vi "VisionTrackingLabVeiwCode.vi"(0 "Image In":T1, 7 "error in":errorcluster) -> (20 "Image Out":T1, 27 "error out":errorcluster)   [LabVIEW 2016]
uses:
  <vilib>/vision/Image Controls.llb/IMAQ Image.ctl
  <vilib>/vision/Tracking.llb/IMAQ Object Tracking SessionType.ctl
  <vilib>/vision/Vision Assistant Utils.llb/IVA Object Tracking - Init Function.ctl
  <vilib>/vision/NI_Vision_Development_Module.lvlib
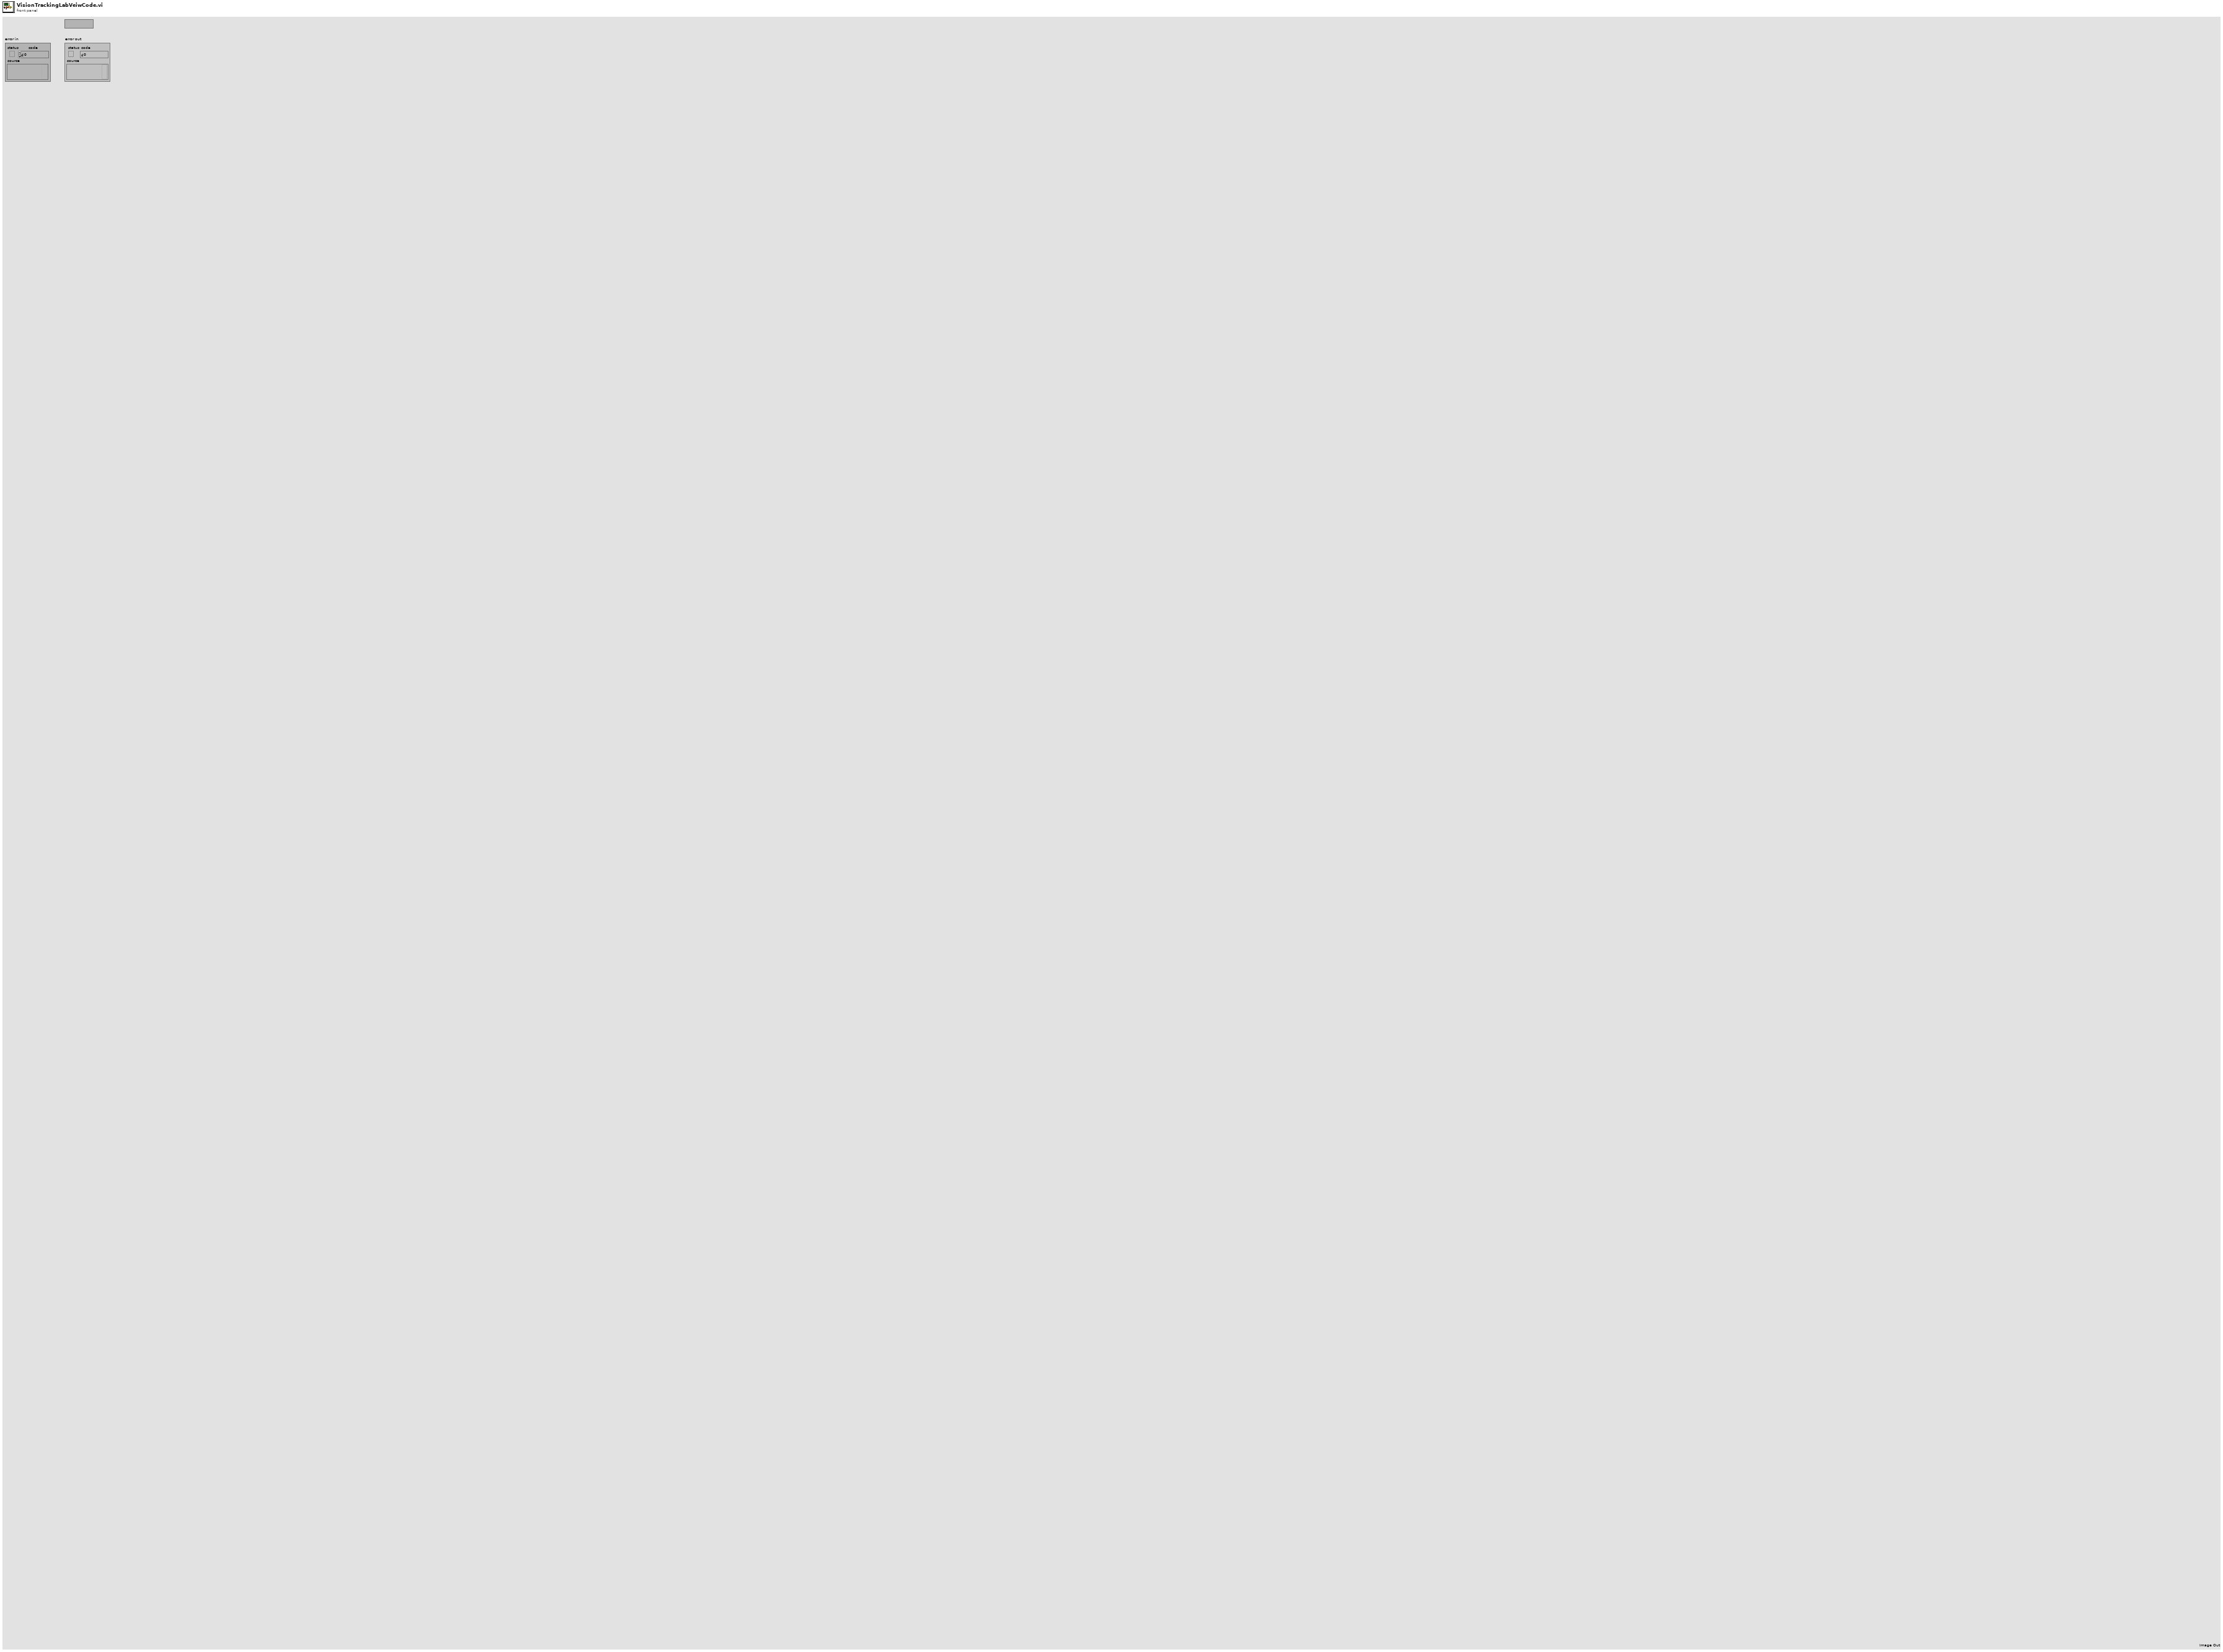
[diagram p1: front panel]
types:
  T1 = typedef "IMAQ Image.ctl" = refnum<image>
  T2 = cluster{"Number of Histogram Bins":i32, "Blending Parameter (%)":dbl, "Max Scale Change (%)":dbl, "Max Rotation Change":dbl, "Max Shape Change (%)":dbl, "Maximum Iterations":i32}
  T3 = typedef "IVA Object Tracking - Init Function.ctl" = enum16{"Init", "Get", "Set"}
  T4 = cluster{"Initial Position":cluster{"Source":enum16{"Constant", "Measure"}, "Point ID":cluster{"GUID":string, "Index":i32}, "Point":cluster{"x":sgl, "y":sgl}}, "Initial Angle":cluster{"Source":enum16{"Constant", "Measure"}, "Measure ID":cluster{"GUID":string, "Index":i32}, "Value":dbl}}[]
  T5 = typedef "IMAQ Object Tracking SessionType.ctl" = i32
  T6 = typedef "Image Type" = u32
  T7 = cluster{"Global Rectangle":i32[], "Contours":cluster{"ID":enum32{"External", "Internal"}, "Type":u32, "Coordinates":i32[]}[]}
  T8 = cluster{"Brightness":sgl, "Contrast":sgl, "Gamma":sgl}
  T9 = cluster{"Position":cluster{"x":sgl, "y":sgl}, "Angle":sgl, "Scale":sgl, "Score":sgl, "Bounding Box":cluster{"x":sgl, "y":sgl}[]}[]
  T10 = cluster{"Number of Histogram Bins":i32, "Blending Parameter (%)":dbl, "Maximum Iterations":i32}
  T11 = typedef "IMAQ Object Tracking Session.ctl" = refnum<k20>
  T12 = cluster{"Source":enum16{"Constant", "Measure"}, "Point ID":cluster{"GUID":string, "Index":i32}, "Point":cluster{"x":sgl, "y":sgl}}
  T13 = cluster{"Source":enum16{"Constant", "Measure"}, "Measure ID":cluster{"GUID":string, "Index":i32}, "Value":dbl}
  T14 = cluster{"Label":string, "Score":i32, "Angle":dbl, "Location":cluster{"X":dbl, "Y":dbl}, "Bounding Box":cluster{"X":dbl, "Y":dbl}[], "Object Found?":bool}[]
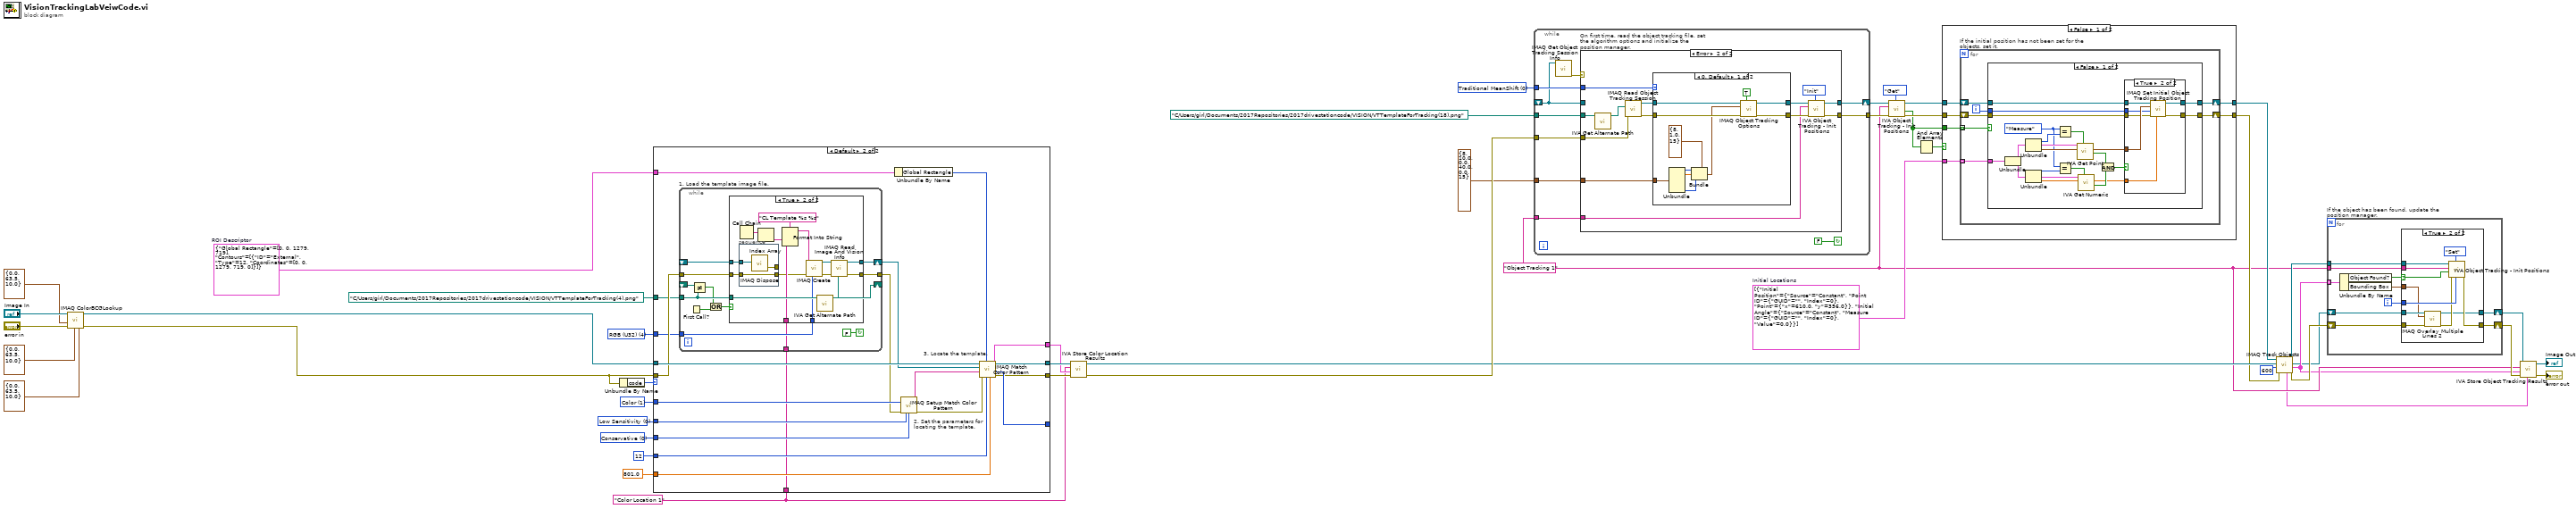
[diagram p0: block diagram]
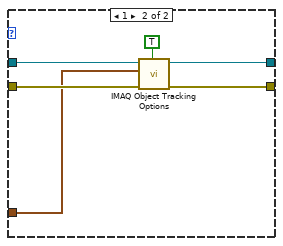
[diagram p7: hidden frame]
diagram:
  w6 = "Object Tracking 1" ("Step Name")
  w21 = T4 [{"Initial Position"={"Source"=enum."Constant", "Point ID"={"GUID"="", "Index"=0}, "Point"={"x"=610.0, "y"=356.0}}, "Initial Angle"={"Source"=enum."Constant", "Measure ID"={"GUID"="", "Index"=0}, "Value"=0.0}}]  # Initial Locations
  w23 = T5 0 items=["Traditional MeanShift", "Shape Adapted MeanShift"] ("Algorithm")
  w26 = "Color Location 1" ("Step Name")
  w34 = T6 4 items=["Grayscale (U8)", "Grayscale (I16)", "Grayscale (SGL)", "Complex (CSG)", "RGB (U32)", "HSL (U32)", "RGB (U64)"] ("Image Type")
  w36 = u32 0 items=["Conservative", "Balance", "Aggressive", "Very Aggressive"] ("Search Strategy")
  w37 = u32 0 items=["Low Sensitivity", "Medium Sensitivity", "High Sensitivity"] ("Color Sensitivity")
  w38 = u32 1 items=["Color and Shape", "Color", "Shape"] ("Match Feature Mode")
  w33 = T7 {"Global Rectangle"=[0, 0, 1279, 719], "Contours"=[{"ID"=enum."External", "Type"=12, "Coordinates"=[0, 0, 1279, 719, 0]}]}  # ROI Descriptor
  n1 = call "IMAQ ColorBCGLookup"("Blue BCG Values"=T8 {"Brightness"=0.0, "Contrast"=63.5, "Gamma"=10.0}, "Green BCG Values"=T8 {"Brightness"=0.0, "Contrast"=63.5, "Gamma"=10.0}, "error in (no error)"="error in", "Red BCG Values"=T8 {"Brightness"=0.0, "Contrast"=63.5, "Gamma"=10.0}, "Image Src"="Image In") -> ("error out"=w44:errorcluster, "Image Dst Out"=w32:T1)  [unwired: 2 in, 3 out]
  n2 = Unbundle By Name(w44) -> ("code"=w31:i32)
  n3 = case shown="Default" w31 {
    tunnel: sgl 801.0 ("Minimum Match Score") -> [_ w66]
    tunnel: 12 ("Number of Matches Requested") -> [_ w65]
    tunnel: [_ w64] -> _
    tunnel: w38 -> [_ w63]
    tunnel: w37 -> [_ w62]
    tunnel: w36 -> [_ w61]
    tunnel: path "C:/Users/girl/Documents/2017Repositories/2017drivestationcode/VISION/VTTemplateForTracking(4).png" ("File Path") -> [_ w53]
    tunnel: w34 -> [_ w52]
    tunnel: w44 -> [_ w54]
    tunnel: w33 -> [_ w58]
    tunnel: [_ w56] -> w27
    tunnel: w32 -> [w47 w55]
    tunnel: [w47 w55] -> w28
    tunnel: [_ w49] -> w29
    tunnel: w26 -> [_ w48]
    frame -1074396199, -1074396198 {
      # "Discard Coordinate System Error"
    }
    frame Default {
      # "3. Locate the template."
      # "2. Set the parameters for\nlocating the template."
      n4 = while "1. Load the template image file." {
        shift-right: [w78] -> w51
        shift-left: _ -> [w77]
        tunnel: [w75] -> w50
        tunnel: w54 -> [w74]
        tunnel: w53 -> [w70]
        tunnel: w52 -> [w73]
        tunnel: w48 -> [w72]
        shift-right: [w70] -> _
        shift-left: _ -> [w71]
        stop <- FALSE continue-if-true
        n5 = First Call?() -> (First Call?: T/F=w69:bool)
        n6 = Not Equal?(x=w71, y=w70) -> (x != y?=w68:bool)
        n7 = Or(x=w68, y=w69) -> (x .or. y?=w67:bool)
        n8 = case shown="True" w67 {
          tunnel: [w80 w93] -> w78
          tunnel: w77 -> [w80 w85]
          tunnel: [w79 w90] -> w75
          tunnel: w74 -> [w79 w84]
          tunnel: w73 -> [_ w89]
          tunnel: w72 -> [_ w86]
          tunnel: w70 -> [_ w82]
          frame False {
          }
          frame True {
            n9 = Call Chain() -> (call chain=w88:string[])
            n10 = stacked-sequence {
              tunnel: w85 -> [w98]
              tunnel: w84 -> [w97]
              tunnel: [w97] -> w83
              tunnel: [w96] -> _
              frame #0 {
                n11 = call "IMAQ Dispose"("Image"=w98) -> ("error out"=w96:errorcluster)  [unwired: 2 in, 3 out]
              }
            }
            n12 = Index Array(array=w88) -> (element=w87:string)  [unwired: 1 in]
            n13 = Format Into String(format string="CL Template %s %s" ("Image Name"), w87, w86) -> (resulting string=w95:string)  [unwired: 2 in, 1 out]
            n14 = call "IMAQ Create"("Image Name"=w95, "Image Type"=w89, "error in (no error)"=w83) -> ("New Image"=w92:T1, "error out"=w91:errorcluster)  [unwired: 1 in, 1 out]
            n15 = call <vilib>:"IVA Get Alternate Path.vi"("Path In"=w82) -> ("Path Out"=w81:path)  [unwired: 10 out]
            n16 = call "IMAQ Read Image And Vision Info"("File Path"=w81, "error in (no error)"=w91, "Image"=w92) -> ("error out"=w90:errorcluster, "Image Out"=w93:T1)  [unwired: 1 in, 6 out]
          }
        }
      }
      n17 = Unbundle By Name(w58) -> ("Global Rectangle"=w57:i32[])
      n18 = call "IMAQ Setup Match Color Pattern"("Match Feature Mode"=w63, "error in (no error)"=w50, "Color Sensitivity"=w62, "Search Strategy"=w61) -> ("Match Color Pattern Setup Data"=w60:string, "error out"=w59:errorcluster)  [unwired: 5 in, 5 out]
      n19 = call "IMAQ Match Color Pattern"("Minimum Match Score"=w66, "Number of Matches Requested"=w65, "Optional Rectangle"=w57, "error in (no error)"=w59, "Match Color Pattern Setup Data"=w60, "Template Image"=w51, "Image"=w55) -> ("error out"=w49:errorcluster, "Number of Matches"=w64:i32, "Matches"=w56:T9)  [unwired: 2 out]
    }
  }
  n20 = call <vilib>:"IVA Store Color Location Results.vi"("error in (no error)"=w29, "Matches"=w27, "Step Name"=w26, "Image in"=w28) -> ("error out"=w30:errorcluster, "Image dup"=w24:T1)  [unwired: 6 out]
  n21 = while {
    shift-right: [w108] -> w19
    shift-left: _ -> [w99]
    tunnel: path "C:/Users/girl/Documents/2017Repositories/2017drivestationcode/VISION/VTTemplateForTracking(18).png" ("Tracking Session File Path") -> [w106]
    tunnel: w30 -> [w105]
    tunnel: w23 -> [w104]
    tunnel: [w103] -> w16
    tunnel: T2 {"Number of Histogram Bins"=8, "Blending Parameter (%)"=10.0, "Max Scale Change (%)"=0.0, "Max Rotation Change"=40.0, "Max Shape Change (%)"=0.0, "Maximum Iterations"=15} ("Options") -> [w102]
    tunnel: w6 -> [w101]
    stop <- FALSE continue-if-true
    n22 = call "IMAQ Get Object Tracking Session Info"("Object Tracking Session In"=w99) -> ("error out"=w100:errorcluster)  [unwired: 1 in, 9 out]
    n23 = case "On first time, read the object tracking file, set the algorithm options and initialize the position manager." shown="Error" w100 {
      tunnel: [w110 w115] -> w108
      tunnel: w99 -> [w110 _]
      tunnel: w106 -> [_ w123]
      tunnel: w105 -> [w109 w121]
      tunnel: w104 -> [_ w120]
      tunnel: [w109 w114] -> w103
      tunnel: w102 -> [_ w117]
      tunnel: w101 -> [_ w111]
      frame No Error {
      }
      frame Error {
        n24 = call <vilib>:"IVA Get Alternate Path.vi"("Path In"=w123) -> ("Path Out"=w122:path)  [unwired: 10 out]
        n25 = call "IMAQ Read Object Tracking Session"("error in (no error)"=w121, "Object Tracking Session File Path"=w122) -> ("error out"=w118:errorcluster, "Object Tracking Session Out"=w119:T11)  [unwired: 1 in, 7 out]
        n26 = case shown="0, Default" w120 {
          tunnel: w119 -> [w134 w140]
          tunnel: [w133 w139] -> w116
          tunnel: w118 -> [w132 w138]
          tunnel: [w131 w137] -> w113
          tunnel: w117 -> [w130 w136]
          frame 0, Default {
            n27 = Unbundle(w130) -> ("Number of Histogram Bins"=w129:i32, "Blending Parameter (%)"=w128:dbl, "Maximum Iterations"=w124:i32)  [unwired: 3 out]
            n28 = Bundle(cluster=T10 {"Number of Histogram Bins"=8, "Blending Parameter (%)"=1.0, "Maximum Iterations"=15} ("Mean Shift Options in"), "Number of Histogram Bins"=w129, "Blending Parameter (%)"=w128, "Maximum Iterations"=w124) -> (w127:T10)
            n29 = call-poly "IMAQ Object Tracking Options"("Get/Set (Get)"=TRUE, "error in (no error)"=w132, "Mean Shift Options in"=w127, "Object Tracking Session In"=w134) -> ("error out"=w131:errorcluster, "Object Tracking Session Out"=w133:T11)  [unwired: 1 in, 5 out]
          }
          frame 1 {
            n30 = call-poly "IMAQ Object Tracking Options"("Get/Set (Get)"=TRUE, "error in (no error)"=w138, "Shape Adapted Options in"=w136, "Object Tracking Session In"=w140) -> ("error out"=w137:errorcluster, "Object Tracking Session Out"=w139:T11)  [unwired: 2 in, 4 out]
          }
        }
        n31 = call <vilib>:"IVA Object Tracking - Init Positions.vi"("Function"=IVA_Object_Tracking_-_Init_Function."Init", "error in (no error)"=w113, "Process ID"=w111, "Object Tracking Session In"=w116) -> ("error out"=w114:errorcluster, "Object Tracking Session dup"=w115:T11)  [unwired: 2 in, 4 out]
      }
    }
  }
  n32 = call <vilib>:"IVA Object Tracking - Init Positions.vi"("Function"=IVA_Object_Tracking_-_Init_Function."Get", "error in (no error)"=w16, "Process ID"=w6, "Object Tracking Session In"=w19) -> ("error out"=w15:errorcluster, "Init Values Out"=w13:bool[], "Object Tracking Session dup"=w18:T11)  [unwired: 2 in, 3 out]
  n33 = And Array Elements(Boolean array=w13) -> (logical AND=w14:bool)
  n34 = case shown="False" w14 {
    tunnel: w21 -> [w146 _]
    tunnel: [w145 w188] -> w20
    tunnel: w18 -> [w144 w188]
    tunnel: w15 -> [w143 w187]
    tunnel: w13 -> [w142 _]
    tunnel: [w141 w187] -> w12
    frame False {
      n35 = for "If the initial position has not been set for the objects, set it." {
        tunnel: w146 -> [w152] mode=indexing
        shift-right: [w150] -> w145
        shift-left: w144 -> [w153]
        shift-right: [w147] -> w141
        shift-left: w143 -> [w149]
        tunnel: w142 -> [w148] mode=indexing
        i -> [w151]
        n36 = case shown="False" w148 {
          tunnel: w153 -> [w175 w186]
          tunnel: w152 -> [w174 _]
          tunnel: w151 -> [w158 _]
          tunnel: [w156 w186] -> w150
          tunnel: w149 -> [w155 w185]
          tunnel: [w154 w185] -> w147
          frame False {
            w164 = enum16{"Constant", "Measure"}."Measure" ("Source")
            n37 = Unbundle(w174) -> ("Initial Position"=w173:T12, "Initial Angle"=w172:T13)
            n38 = Unbundle(w173) -> ("Source"=w167:enum16{"Constant", "Measure"}, "Point ID"=w171:cluster{"GUID":string, "Index":i32}, "Point"=w170:cluster{"x":sgl, "y":sgl})
            n39 = Unbundle(w172) -> ("Source"=w165:enum16{"Constant", "Measure"}, "Measure ID"=w169:cluster{"GUID":string, "Index":i32}, "Value"=w168:dbl)
            n40 = Equal?(x=w164, y=w167) -> (x = y?=w166:bool)
            n41 = Equal?(x=w164, y=w165) -> (x = y?=w163:bool)
            n42 = call <vilib>:"IVA Get Point.vi"("Point Source"=w166, "Point in"=w170, "Point ID"=w171) -> ("Available?"=w162:bool, "Point out"=w159:cluster{"x":sgl, "y":sgl})  [unwired: 1 in, 6 out]
            n43 = call <vilib>:"IVA Get Numeric.vi"("Source"=w163, "Numeric in"=w168, "Result ID"=w169) -> ("Available?"=w161:bool, "Numeric out"=w157:dbl)  [unwired: 1 in, 6 out]
            n44 = And(x=w162, y=w161) -> (x .and. y?=w160:bool)
            n45 = case shown="True" w160 {
              tunnel: w175 -> [w177 w184]
              tunnel: w159 -> [_ w183]
              tunnel: w158 -> [_ w182]
              tunnel: w157 -> [_ w178]
              tunnel: [w177 w181] -> w156
              tunnel: w155 -> [w176 w180]
              tunnel: [w176 w179] -> w154
              frame False {
              }
              frame True {
                n46 = call "IMAQ Set Initial Object Tracking Position"("Initial Angle"=w178, "error in (no error)"=w180, "Object Index"=w182, "Position"=w183, "Object Tracking Session In"=w184) -> ("error out"=w179:errorcluster, "Object Tracking Session Out"=w181:T11)  [unwired: 5 out]
              }
            }
          }
          frame True {
          }
        }
      }
    }
    frame True {
    }
  }
  n47 = call "IMAQ Track Objects"("error in (no error)"=w12, "Minimum Score"=600, "Image"=w24, "Object Tracking Session In"=w20) -> ("error out"=w11:errorcluster, "Objects (pixel)"=w5:T14, "Image (duplicate)"=w2:T1, "Object Tracking Session Out"=w10:T11, "Objects (real-world)"=w4:T14)  [unwired: 3 out]
  n48 = for "If the object has been found, update the position manager." {
    tunnel: w5 -> [w198] mode=indexing
    tunnel: w6 -> [w197]
    shift-right: [w194] -> w8
    shift-left: w11 -> [w191]
    tunnel: w10 -> [w196]
    shift-right: [w190] -> w1
    shift-left: w2 -> [w192]
    i -> [w193]
    n49 = Unbundle By Name(w198) -> ("Object Found?"=w195:bool, "Bounding Box"=w189:cluster{"X":dbl, "Y":dbl}[])
    n50 = case shown="True" w195 {
      selector: w195 -> [_ w208]
      tunnel: w197 -> [_ w210]
      tunnel: w196 -> [_ w209]
      tunnel: [w200 w207] -> w194
      tunnel: w193 -> [_ w206]
      tunnel: w192 -> [w199 w205]
      tunnel: w191 -> [w200 w203]
      tunnel: [w199 w202] -> w190
      tunnel: w189 -> [_ w201]
      frame False {
      }
      frame True {
        n51 = call "IMAQ Overlay Multiple Lines 2"("Image"=w205, "Line End Points"=w201, "error in (no error)"=w203) -> ("Image Out"=w202:T1, "error out"=w204:errorcluster)  [unwired: 11 in]
        n52 = call <vilib>:"IVA Object Tracking - Init Positions.vi"("Index"=w206, "Function"=IVA_Object_Tracking_-_Init_Function."Set", "error in (no error)"=w204, "Value"=w208, "Process ID"=w210, "Object Tracking Session In"=w209) -> ("error out"=w207:errorcluster)  [unwired: 5 out]
      }
    }
  }
  n53 = call <vilib>:"IVA Store Object Tracking Results.vi"("Objects (real-world)"=w4, "error in (no error)"=w8, "Objects (pixel)"=w5, "Step Name"=w6, "Image in"=w1) -> ("error out"=→"error out":errorcluster, "Image dup"=→"Image Out":T1)  [unwired: 5 out]
